vi "Init.vi"(6 "PortCfg":T1={"baud rate (9600)"=9600, "data bits (8)"=8, "stop bits (10: 1 bit)"=10, "termination char\n(0xA = '\\n' = LF) "=10, "parity (0:none)"=enum."None", "timeout (10sec)"=10000, "Enable Termination\nChar (T)"=TRUE, "flow control (0:none)"=0} {"flow control (0:none)" items=["None", "XON/XOFF", "RTS/CTS", "XON/XOFF & RTS/CTS", "DTR/DSR", "XON/XOFF & DTR/DSR"]; "termination char\n(0xA = '\\n' = LF)" format="%.0x"; "stop bits (10: 1 bit)" items=["1.0"=10, "1.5"=15, "2.0"=20]; "data bits (8)" min=5 max=8 step=1}, 7 "Name":string, 8 "error in":errorcluster, 10 "Port":refnum<visa-resource-name>, 11 "CN79000 in":refnum<class "CN79000.lvclass">) -> (0 "error out":errorcluster, 3 "CN79000 out":refnum<class "CN79000.lvclass">)   [LabVIEW 2011, in "CN79000.lvclass"]
doc: "Initialize communication with a serial port. Open the port and obtain a reference to a semaphore that will be used to prevent communication clashes."
uses:
  CN79000.lvclass
  Base/Serial IO.lvclass
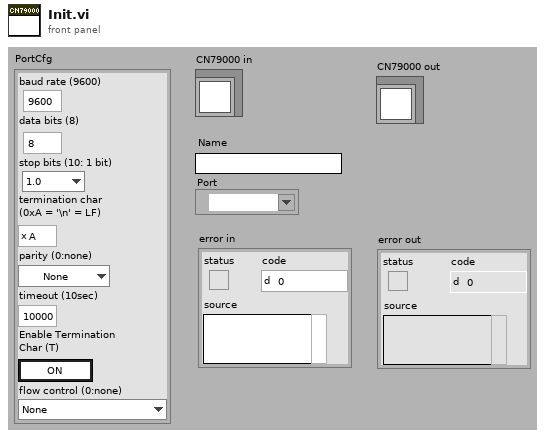
[diagram p1: front panel]
types:
  T1 = cluster{"baud rate (9600)":u32, "data bits (8)":u16, "stop bits (10: 1 bit)":u16, "termination char\n(0xA = '\\n' = LF) ":u8, "parity (0:none)":enum16{"None", "Odd", "Even", "Mark", "Space"}, "timeout (10sec)":u32, "Enable Termination\nChar (T)":bool, "flow control (0:none)":u16}
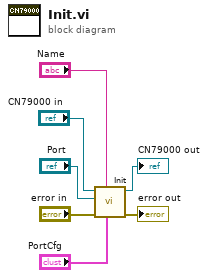
[diagram p0: block diagram]
diagram:
  n1 = call-parent "Init.vi"("PortCfg"="PortCfg", "Name"="Name", "error in"="error in", "Port"="Port", "Serial IO in"="CN79000 in") -> ("error out"=→"error out":errorcluster, "Serial IO out"=→"CN79000 out":refnum<class "CN79000.lvclass">)  [unwired: 5 in]
